vi "Extract Test Result of Analog Test with Match Pattern.vi"() -> ()   [LabVIEW 2020]
panel:
  out "Offset Past Match":i32[](array[numeric])
  out "Numeric":i32
  out "Strings":string[](array[string])
  out "Numbers":string[](array[string])
  out "Numbers":dbl[](array[numeric])
  in  "Stop Button":bool
  in  "String":string="one 2 -3 4.0 5.5"
  # "OverView :"
  # "Note :"
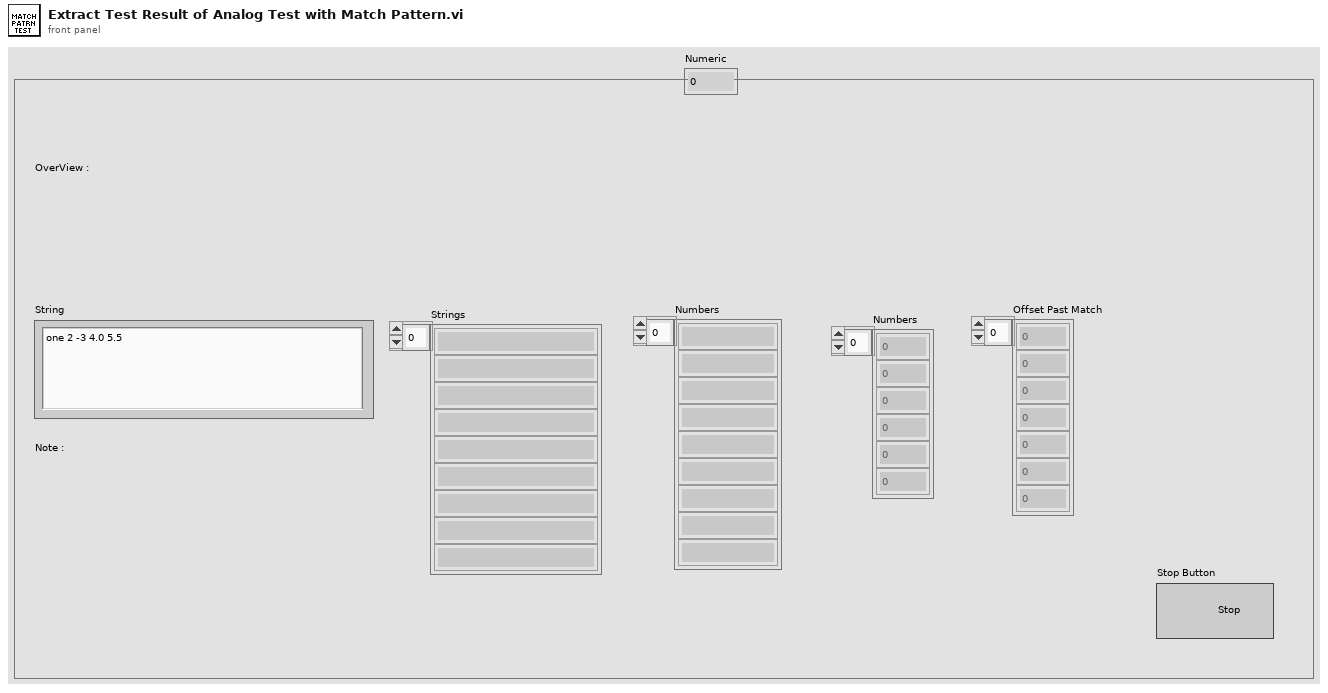
[diagram p1: front panel]
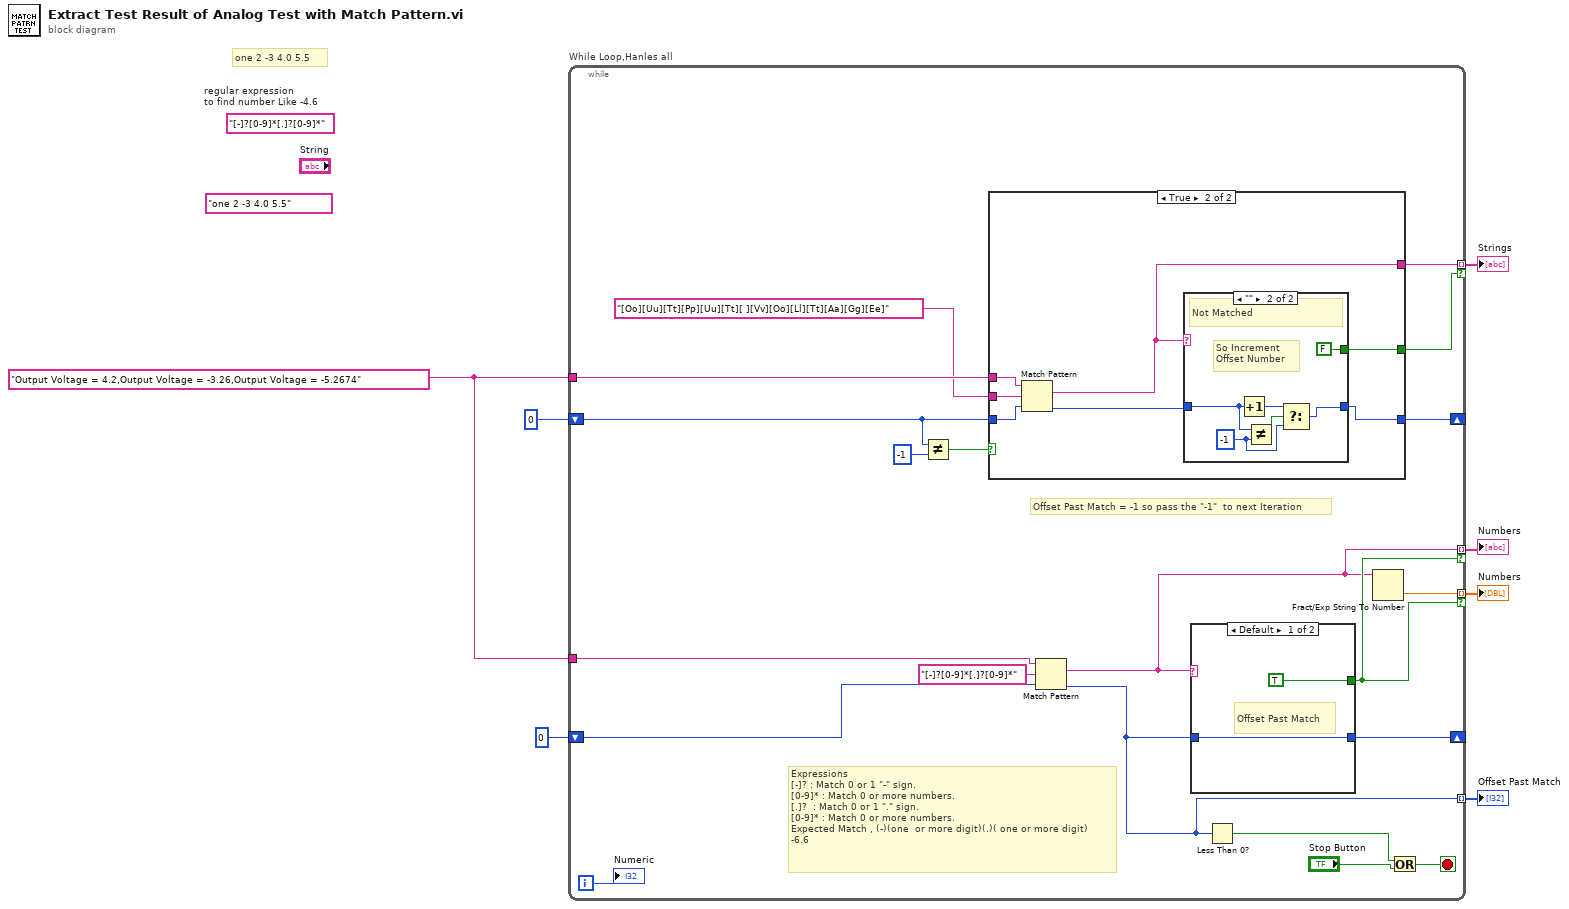
[diagram p0: block diagram]
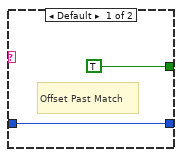
[diagram p3: hidden frame]
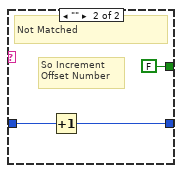
[diagram p4: hidden frame]
diagram:
  (unwired) "[-]?[0-9]*[.]?[0-9]*"  # regular expression  to find number Like -4.6
  w3 = "Output Voltage = 4.2,Output Voltage = -3.26,Output Voltage = -5.2674" ("String")
  (unwired) "one 2 -3 4.0 5.5" ("String")
  # "one 2 -3 4.0 5.5"
  n1 = while "While Loop,Hanles all" {
    tunnel: w3 -> [w19]
    tunnel: [w27] -> w6 mode=indexing if=w21
    shift-right: [w9] -> _
    shift-left: 0 -> [w26]
    tunnel: [w20] -> w5 mode=indexing if=w21
    shift-right: [w10] -> _
    shift-left: 0 -> [w13]
    tunnel: [w17] -> w2 mode=indexing if=w16
    tunnel: w3 -> [w15]
    tunnel: [w8] -> w1 mode=indexing
    i -> [w11]
    stop <- w23 stop-if-true
    # "Offset Past Match = -1 so pass the \"-1\"  to next Iteration"
    # "Expressions\n[-]? : Match 0 or 1 \"-\" sign.\n[0-9]* : Match 0 or more numbers.\n[.]?  : Match 0 or 1 \".\" sign.\n[0-9]* : Match 0 or more numbers.\nExpected Match , (-)(one  or more digit)(.)( one or more digit)\n-6.6"
    n2 = Not Equal?(x=w13, y=-1) -> (x != y?=w14:bool)
    n3 = case shown="True" w14 {
      tunnel: w19 -> [_ w35]
      tunnel: "[Oo][Uu][Tt][Pp][Uu][Tt][ ][Vv][Oo][Ll][Tt][Aa][Gg][Ee]" ("regular expression") -> [_ w34]
      tunnel: w13 -> [w28 w33]
      tunnel: [w28 w31] -> w10
      tunnel: [_ w30] -> w17
      tunnel: [_ w29] -> w16
      frame False {
        # "Whole Sting Searched"
      }
      frame True {
        n4 = Match Pattern(string=w35, regular expression=w34, offset (0)=w33) -> (match substring=w30:string, offset past match=w32:i32)  [unwired: 2 out]
        n5 = case shown="\"\"" w30 {
          tunnel: w32 -> [w37 w39]
          tunnel: [w37 w41] -> w31
          tunnel: [TRUE FALSE] -> w29
          frame Default {
            # "Offset Past Match"
          }
          frame "" {
            w38 = -1 ("y")
            # "So Increment \nOffset Number"
            # "Not Matched"
            n6 = Increment(x=w39) -> (x+1=w42:i32)
            n7 = Not Equal?(x=w39, y=w38) -> (x != y?=w40:bool)
            n8 = Select(t=w42, s=w40, f=w38) -> (s? t:f=w41:i32)
          }
        }
      }
    }
    n9 = Match Pattern(string=w15, regular expression="[-]?[0-9]*[.]?[0-9]*", offset (0)=w26) -> (match substring=w20:string, offset past match=w8:i32)  [unwired: 2 out]
    n10 = case shown="Default" w20 {
      tunnel: w8 -> [w45 w48]
      tunnel: [w45 w47] -> w9
      tunnel: [TRUE FALSE] -> w21
      frame Default {
        # "Offset Past Match"
      }
      frame "" {
        # "So Increment \nOffset Number"
        # "Not Matched"
        n11 = Increment(x=w48) -> (x+1=w47:i32)
      }
    }
    n12 = Less Than 0?(x=w8) -> (x < 0?=w22:bool)
    n13 = Fract/Exp String To Number(string=w20) -> (number=w27:dbl)  [unwired: 3 in, 1 out]
    n14 = Or(x=w22, y="Stop Button") -> (x .or. y?=w23:bool)
    "Numeric" <- w11
  }
  "Numbers" <- w6
  "Numbers" <- w5
  "Strings" <- w2
  "Offset Past Match" <- w1
